vi "01TimingSelfTest.vi"(11 "YTESTER测试数据":T1={"Socket(From1)"=1, "SN"=refnum, "StopFlagRef"=refnum, "YT System Queue"=refnum}) -> (3 "YTESTER结论":T2)   [LabVIEW 2017]
doc: "VIDescription="
uses:
  YtCommon.lvlibp/yt`Step StepBaseInput.ctl
  YtCommon.lvlibp/yt`Step StepResult.ctl
  YtCommon.lvlibp/yt`Step TestData.ctl
  YtCommon.lvlibp/yt`Step System Queue.ctl
  d11f19f8-4d98-430b-8262-6558d64bdea2.vi
  <vilib>/Utility/error.llb/Clear Errors.vi
  YtCommon.lvlibp/yt`varSystemlib IO Read Variable.vi
  YtCommon.lvlibp
panel:
  in  "YTESTER开放参数":T4={"YTESTER_BaseInput"={"isTest"=FALSE, "isSkip"=FALSE, "StepName"="重入异步·自动测试", "OnPass"=enum."Next", "OnFail"=enum."Next", "ReTestNumber"=0.0}, "定时触发自动测试(>0.5s)"=3.0}
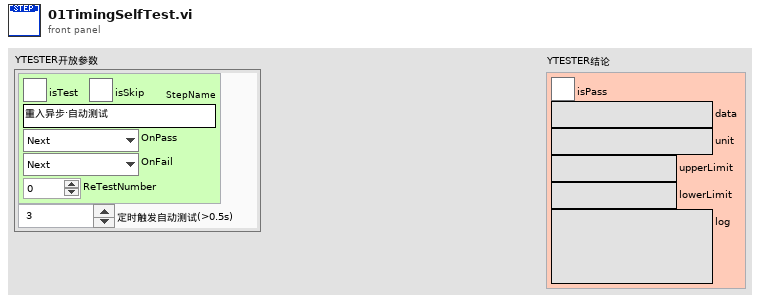
[diagram p1: front panel]
types:
  T1 = typedef "YtCommon.lvlibp/yt`Step TestData.ctl" = cluster{"Socket(From1)":i32, "SN":refnum<notifier>, "StopFlagRef":refnum<notifier>, "YT System Queue":refnum<queue>}
  T2 = typedef "YtCommon.lvlibp/yt`Step StepResult.ctl" = cluster{"isPass":bool, "data":string, "unit":string, "upperLimit":string, "lowerLimit":string, "log":string}
  T3 = typedef "YtCommon.lvlibp/yt`Step StepBaseInput.ctl" = cluster{"isTest":bool, "isSkip":bool, "StepName":string, "OnPass":enum16{"Next", "ToOVER", "Terminate"}, "OnFail":enum16{"Next", "ToOVER", "Terminate"}, "ReTestNumber":dbl}
  T4 = cluster{"YTESTER_BaseInput":T3, "定时触发自动测试(>0.5s)":dbl}
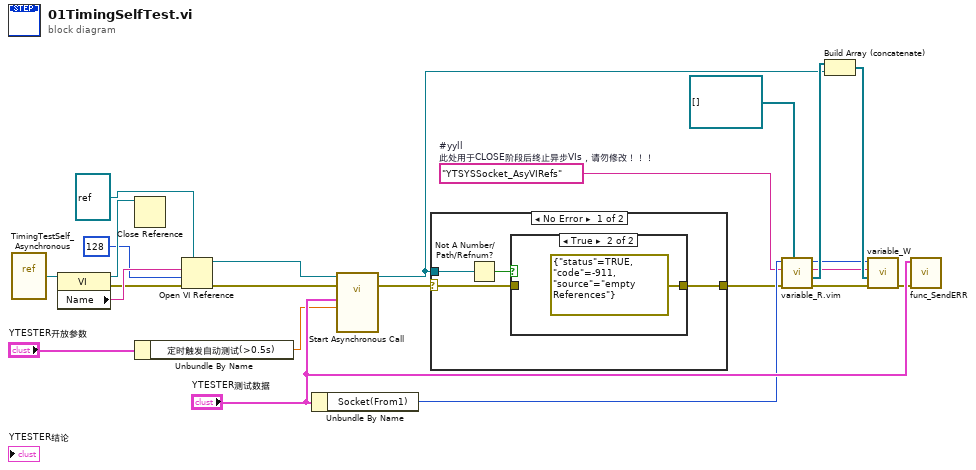
[diagram p0: block diagram]
diagram:
  w6 = "YTSYSSocket_AsyVIRefs"  # #yyll 此处用于CLOSE阶段后终止异步VIs，请勿修改！！！
  n1 = vi-ref "TimingTestSelf_Asynchronous.vi"() -> (w23:refnum<vi>)
  n2 = property class="VI"(reference=w23) -> (reference out=w20:refnum<vi>, error out=w21:errorcluster, "Name"=w22:string)  [unwired: 1 in]
  n3 = Close Reference(reference=w20) -> ()  [unwired: 1 in, 1 out]
  n4 = Unbundle By Name("YTESTER开放参数") -> ("定时触发自动测试(>0.5s)"=w4:dbl)
  n5 = Open VI Reference(type specifier VI Refnum (for type only)=refnum<vi> refnum ("VI引用句柄"), vi path=w22, options=128 ("重入简单异步"), error in (no error)=w21) -> (vi reference=w14:refnum<vi>, error out=w16:errorcluster)  [unwired: 2 in]
  n6 = Unbundle By Name("YTESTER测试数据") -> ("Socket(From1)"=w9:i32)
  n7 = call-by-ref "Start Asynchronous Call"(reference=w14, error in=w16, "定时触发自动测试(s)"=w4, "YTESTER测试数据"="YTESTER测试数据") -> (reference out=w2:refnum<vi>, error out=w3:errorcluster)  [unwired: 10 in]
  n8 = case shown="No Error" w3 {
    selector: w3 -> [w24 w30]
    tunnel: w2 -> [w27 _]
    tunnel: [w25 w30] -> w1
    frame No Error {
      n9 = Not A Number/Path/Refnum?(number/path/refnum=w27) -> (NaN/Path/Refnum?=w26:bool)
      n10 = case shown="True" w26 {
        tunnel: [w28 errorcluster {"status"=TRUE, "code"=-911, "source"="empty References"} ("error IO")] -> w25
        tunnel: w24 -> [w28 _]
        frame False {
        }
        frame True {
        }
      }
    }
    frame Error {
    }
  }
  n11 = call "variable_R.vim"("type"=refnum<vi>[] [] ("reference"), "error in"=w1, "待获取变量名称"=w6, "函数池名称"=w9) -> ("error out"=w13:errorcluster, "value"=w11:refnum<vi>[], "待获取变量名out"=w10:string, "函数池名称out"=w8:i32)  [unwired: 3 in, 1 out]
  n12 = Build Array (concatenate)(w11, w2) -> (w12:refnum<vi>[])
  n13 = call "variable_W.vi"("error in (no error)"=w13, "待写入池的输入控件"=w12, "待写入池变量名称"=w10, "函数池名称 in"=w8) -> ("error out"=w5:errorcluster)  [unwired: 5 in, 2 out]
  n14 = call "func_SendERR.vi"("ERR (String\\Errclust)"=w5, "YTESTER测试数据 in"="YTESTER测试数据") -> ()  [unwired: 9 in, 1 out]
